vi "Read HiPOT Channel.vi"(8 "error in (no error)":errorcluster, 11 "HiPOT Channel configuration":refnum<class "HiPOT Channel configuration.lvclass">) -> (0 "error out":errorcluster, 2 "HiPOT Channel Setting":T1={"Connection"="None"}, 3 "HiPOT Channel configuration out":refnum<class "HiPOT Channel configuration.lvclass">)   [LabVIEW 2025, in "HiPOT.lvlib" / "HiPOT Channel configuration.lvclass"]
uses:
  HiPOT Channel configuration.lvclass
  HiPOT Channel configuration.lvclass/HiPOT Channel configuration.ctl
  HiPOT Channel Setting.ctl
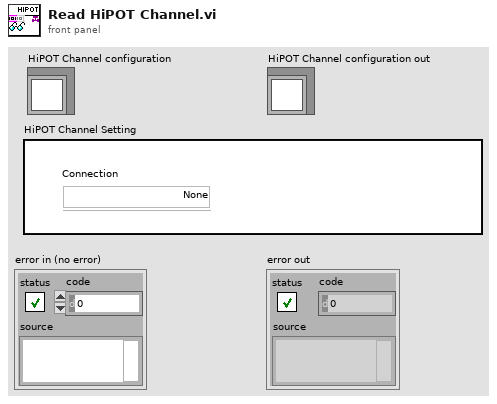
[diagram p1: front panel]
types:
  T1 = typedef "HiPOT.lvlib/HiPOT Channel configuration.lvclass/HiPOT Channel Setting.ctl" = cluster{"Connection":string}
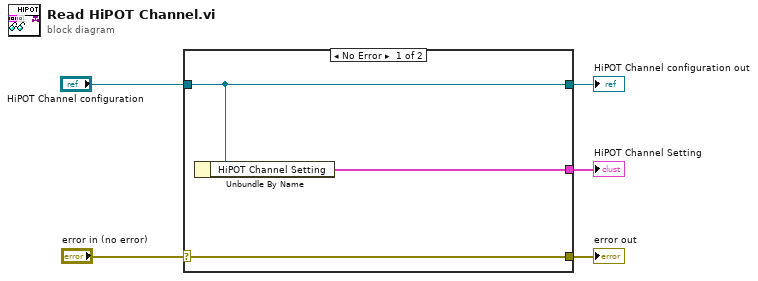
[diagram p0: block diagram]
diagram:
  n1 = case shown="No Error" "error in (no error)" {
    selector: "error in (no error)" -> [w8 w9]
    tunnel: [w8 w9] -> w4
    tunnel: [w7 w10] -> w2
    tunnel: "HiPOT Channel configuration" -> [w7 w10]
    tunnel: [w6 _] -> w1
    frame No Error {
      n2 = Unbundle By Name(w7) -> ("HiPOT Channel Setting"=w6:T1)
    }
    frame Error {
    }
  }
  "error out" <- w4
  "HiPOT Channel configuration out" <- w2
  "HiPOT Channel Setting" <- w1
